vi "extract_image_and_count_electrons.vi"(0 "Image Q In":T1, 11 "Electron Count Q In":T1) -> (4 "Image Q Out":T1, 13 "error out":errorcluster, 15 "Electron Count Q Out":T1)   [LabVIEW 2023]
uses:
  <vilib>/vision/Image Controls.llb/IMAQ Image.ctl
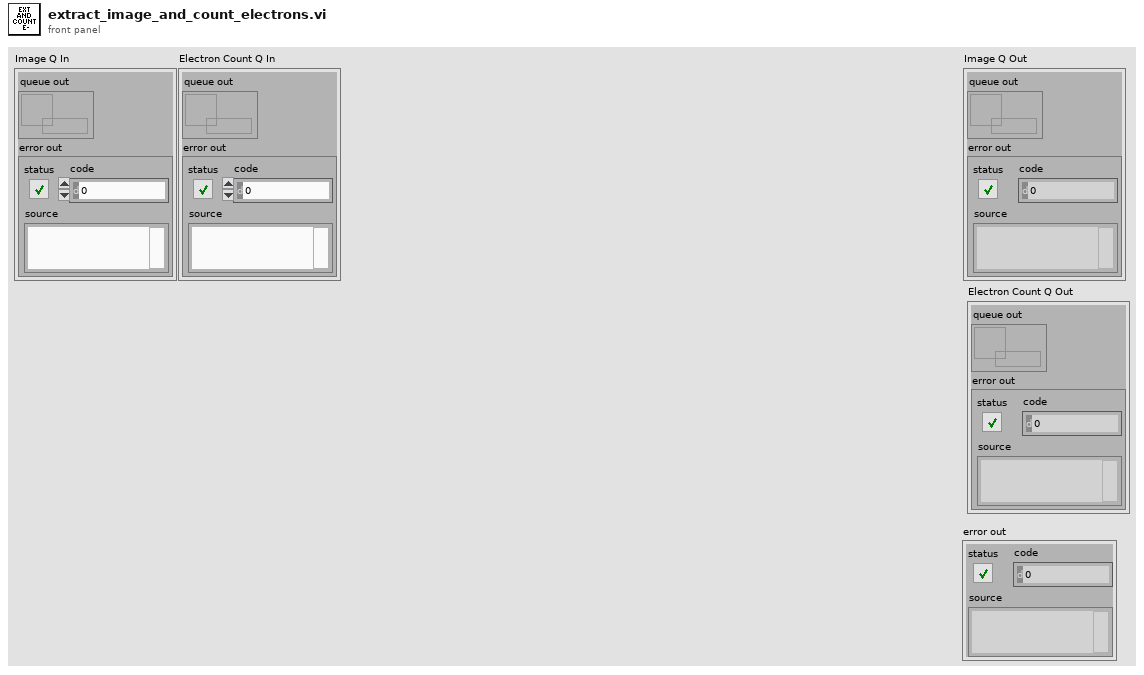
[diagram p1: front panel]
types:
  T1 = cluster{"queue out":refnum<queue>, "error out":errorcluster}
  T2 = typedef "IMAQ Image.ctl" = refnum<image>
  T3 = cluster{"Image Out":T2, "Image Data":cluster{"Actual Width":u32, "Actual Height":u32, "Buffer Number":i32}, "Imaging Variables In":cluster{"Region of interest":i32[], "Number of buffers":u32, "Frame timeout (ms)":u32}}
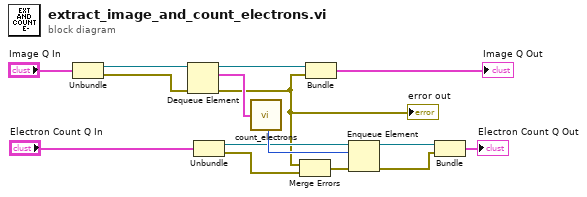
[diagram p0: block diagram]
diagram:
  n1 = Unbundle("Image Q In") -> ("queue out"=w14:refnum<queue>, "error out"=w13:errorcluster)
  n2 = Dequeue Element(queue=w14, error in (no error)=w13) -> (queue out=w12:refnum<queue>, element=w10:T3, error out=w2:errorcluster)  [unwired: 1 in, 1 out]
  "error out" <- w2
  n3 = Unbundle("Electron Count Q In") -> ("queue out"=w7:refnum<queue>, "error out"=w1:errorcluster)
  n4 = call "count_electrons.vi"("Raw Image Data In"=w10) -> ("Electron Counts Out"=w9:i32)  [unwired: 13 in, 1 out]
  n5 = Merge Errors(w2, w1) -> (w3:errorcluster)
  n6 = Bundle("queue out"=w12, "error out"=w2) -> (→"Image Q Out":T1)  [unwired: 1 in]
  n7 = Enqueue Element(queue=w7, element=w9, error in (no error)=w3) -> (queue out=w6:refnum<queue>, error out=w5:errorcluster)  [unwired: 1 in, 1 out]
  n8 = Bundle("queue out"=w6, "error out"=w5) -> (→"Electron Count Q Out":T1)  [unwired: 1 in]
